vi "Read RRT Parameters.vi"(8 "error in (no error)":errorcluster, 11 "Parameters in":refnum<class "Parameters.lvclass">) -> (0 "error out":errorcluster, 2 "RRT Parameters":T1={"threshold"=120.0, "Step"=120.0, "GoalProb"=0.1, "WayPointProb"=0.6} {"WayPointProb" format="%#_13g"; "GoalProb" format="%#_13g"}, 3 "Parameters out":refnum<class "Parameters.lvclass">)   [LabVIEW 2023, in "Parameters.lvclass"]
uses:
  Parameters.lvclass
  Game_class/PathPlanning/Path Planning/RRT/RRTParameters.ctl
  Parameters.lvclass/Parameters.ctl
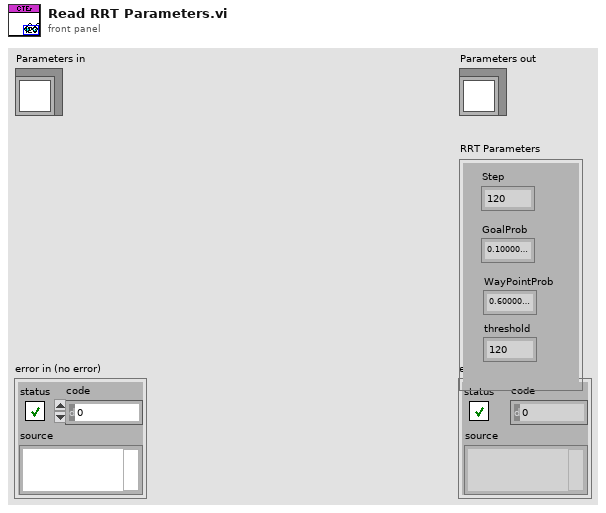
[diagram p1: front panel]
types:
  T1 = typedef "RRTParameters.ctl" = cluster{"threshold":sgl, "Step":sgl, "GoalProb":sgl, "WayPointProb":sgl}
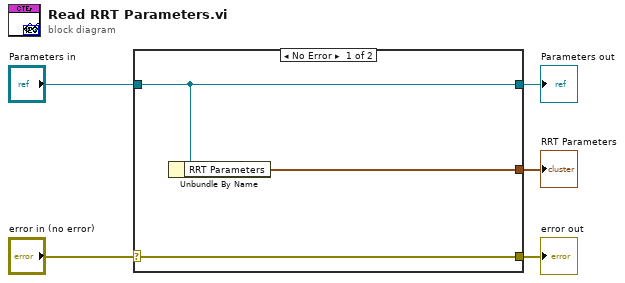
[diagram p0: block diagram]
diagram:
  n1 = case shown="No Error" "error in (no error)" {
    selector: "error in (no error)" -> [w8 w9]
    tunnel: [w8 w9] -> w4
    tunnel: [w7 w10] -> w2
    tunnel: "Parameters in" -> [w7 w10]
    tunnel: [w6 _] -> w1
    frame No Error {
      n2 = Unbundle By Name(w7) -> ("RRT Parameters"=w6:T1)
    }
    frame Error {
    }
  }
  "error out" <- w4
  "Parameters out" <- w2
  "RRT Parameters" <- w1
